vi "Select_Desired_Indicies.vi"(5 "No of averages":i32=1, 7 "Clients time":dbl, 8 "End time":dbl, 9 "Start time":dbl, 10 "Table values":dbl[][](array[numeric]) format="%.2f") -> (0 "Length":i32[](array[numeric]), 1 "End Integer":i32[](array[numeric]), 2 "Start integer":i32[](array[numeric]), 3 "Averaging Times":dbl[](array[numeric]) format="%.2f", 4 "Client leads me by:":dbl, 6 "Total Time":dbl format="%.2f")   [LabVIEW 2010]
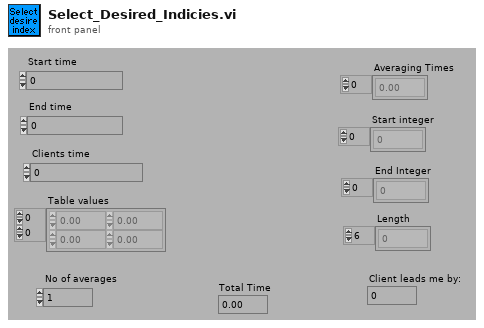
[diagram p1: front panel]
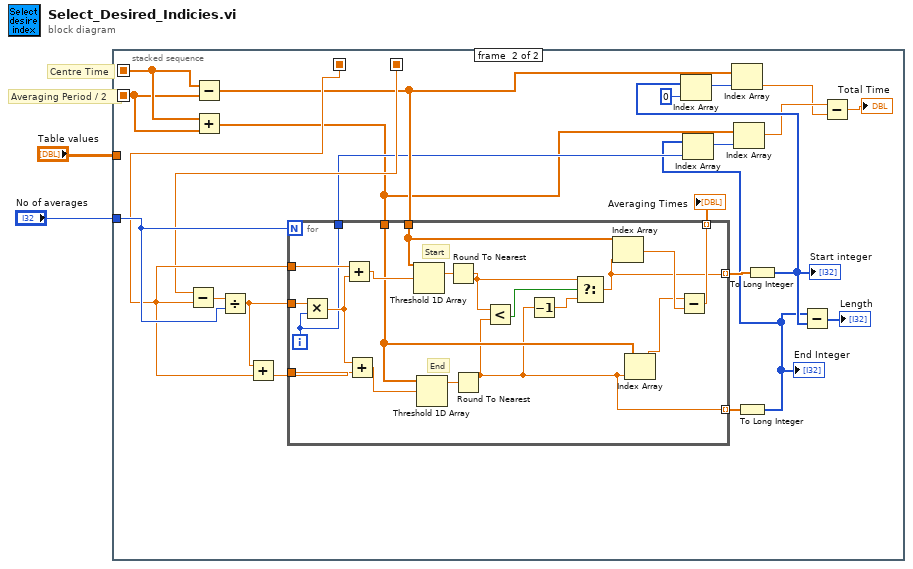
[diagram p0: block diagram]
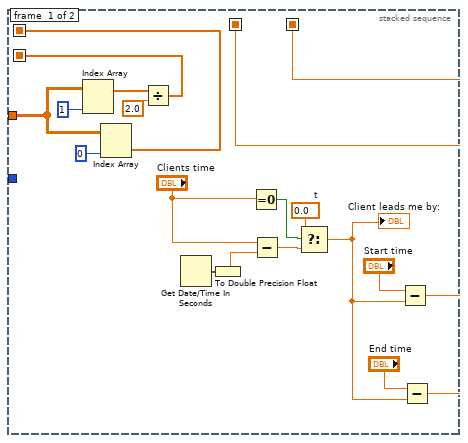
[diagram p2: hidden frame]
diagram:
  # "Averaging Period / 2"
  # "Centre Time"
  n1 = stacked-sequence {
    seq-local: [w8 _] -> [_ w37]
    seq-local: [w12 _] -> [_ w39]
    seq-local: [w13 _] -> [_ w38]
    seq-local: [w4 _] -> [_ w36]
    tunnel: "Table values" -> [w9 _]
    tunnel: "No of averages" -> [_ w40]
    frame #0 {
      w14 = 0.0  # t
      n2 = Index Array(array=w9, index (col)=1) -> (element=w6:dbl[])  [unwired: 1 in]
      n3 = Index Array(array=w9, index (col)=0) -> (element=w8:dbl[])  [unwired: 1 in]
      n4 = Divide(x=w6, y=2.0) -> (x/y=w4:dbl[])
      n5 = Get Date/Time In Seconds() -> (seconds since 1Jan1904=w3:timestamp)
      n6 = To Double Precision Float(number=w3) -> (double precision float=w20:dbl)
      n7 = Equal To 0?(x="Clients time") -> (x = 0?=w15:bool)
      n8 = Subtract(x="Clients time", y=w20) -> (x-y=w16:dbl)
      n9 = Select(t=w14, s=w15, f=w16) -> (s? t:f=w7:dbl)
      "Client leads me by:" <- w7
      n10 = Subtract(x="Start time", y=w7) -> (x-y=w12:dbl)
      n11 = Subtract(x="End time", y=w7) -> (x-y=w13:dbl)
    }
    frame #1 {
      n12 = Subtract(x=w38, y=w39) -> (x-y=w43:dbl)
      n13 = Subtract(x=w37, y=w36) -> (x-y=w28:dbl[])
      n14 = Add(x=w37, y=w36) -> (x+y=w24:dbl[])
      n15 = Divide(x=w43, y=w40) -> (x/y=w42:dbl)
      n16 = Add(x=w42, y=w39) -> (x+y=w41:dbl)
      n17 = for {
        N: w40 -> [_]
        tunnel: w42 -> [w62]
        tunnel: w39 -> [w61]
        tunnel: w41 -> [w59]
        tunnel: w28 -> [w53]
        tunnel: [w45] -> w34 mode=indexing
        tunnel: [w46] -> w33 mode=indexing
        tunnel: w24 -> [w54]
        tunnel: [w50] -> w35 mode=indexing
        tunnel: [w49] -> w26
        i -> [w49]
        # "End"
        # "Start"
        n18 = Multiply(x=w62, y=w49) -> (x*y=w60:dbl)
        n19 = Add(x=w61, y=w60) -> (x+y=w58:dbl)
        n20 = Add(x=w60, y=w59) -> (x+y=w55:dbl)
        n21 = Threshold 1D Array(2:w58, 3:w53) -> (0:w57:dbl)  [unwired: 1 out]
        n22 = Threshold 1D Array(2:w55, 3:w54) -> (0:w56:dbl)  [unwired: 1 out]
        n23 = Round To Nearest(number=w57) -> (nearest integer value=w47:dbl)
        n24 = Round To Nearest(number=w56) -> (nearest integer value=w46:dbl)
        n25 = Less?(x=w47, y=w46) -> (x < y?=w48:bool)
        n26 = Decrement(x=w46) -> (x-1=w44:dbl)
        n27 = Select(t=w47, s=w48, f=w44) -> (s? t:f=w45:dbl)
        n28 = Index Array(array=w53, index=w45) -> (element=w52:dbl)
        n29 = Index Array(array=w54, index=w46) -> (element=w51:dbl)
        n30 = Subtract(x=w51, y=w52) -> (x-y=w50:dbl)
      }
      "Averaging Times" <- w35
      n31 = To Long Integer(number=w33) -> (32bit integer=w25:i32[])
      "End Integer" <- w25
      n32 = Index Array(array=w25, index=w26) -> (element=w27:i32)
      n33 = Index Array(array=w24, index=w27) -> (element=w22:dbl)
      n34 = To Long Integer(number=w34) -> (32bit integer=w30:i32[])
      "Start integer" <- w30
      n35 = Index Array(array=w30, index=0 ("Index")) -> (element=w29:i32)
      n36 = Index Array(array=w28, index=w29) -> (element=w21:dbl)
      n37 = Subtract(x=w25, y=w30) -> (x-y=→"Length":i32[])
      n38 = Subtract(x=w22, y=w21) -> (x-y=→"Total Time":dbl)
    }
  }
